vi "Data Save in File.vi"(4 "Data IN":T1, 7 "Data Save Path":path) -> ()   [LabVIEW 2015]
uses:
  Data Save Typdef.ctl
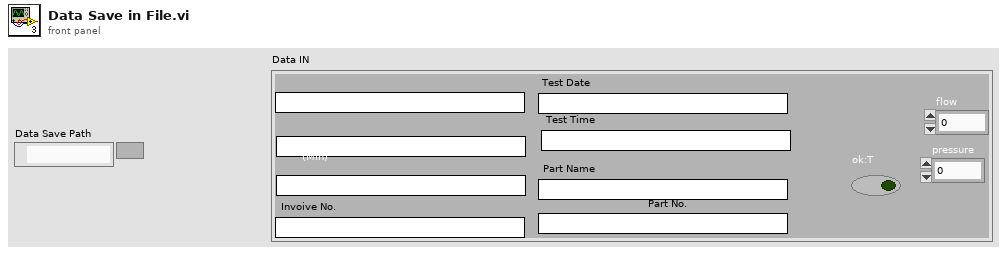
[diagram p1: front panel]
types:
  T1 = typedef "Data Save Typdef.ctl" = cluster{"Pump SI. No.":string, "Operator Name":string, "Batch No.":string, "Invoive No.":string, "Test Date":string, "Test Time":string, "Part Name":string, "Part No.":string, "flow":dbl, "pressure":dbl, "ok:T":bool}
  T2 = enum16{"open", "replace", "create", "open or create", "replace or create", "replace or create with confirmation"}
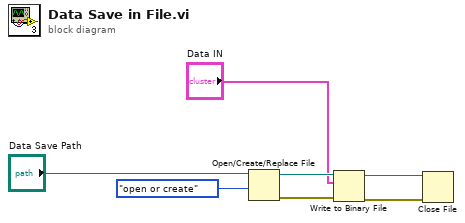
[diagram p0: block diagram]
diagram:
  n1 = Open/Create/Replace File(file path (use dialog)="Data Save Path", operation (0:open)=T2."open or create") -> (refnum out=w5:refnum<file>, error out=w4:errorcluster)  [unwired: 4 in, 1 out]
  n2 = Write to Binary File(file (use dialog)=w5, data="Data IN", error in=w4) -> (refnum out=w7:refnum<file>, error out=w6:errorcluster)  [unwired: 3 in, 1 out]
  n3 = Close File(refnum=w7, error in=w6) -> ()  [unwired: 2 out]
